vi "Object_Create.vi"(0 "reference in":refnum<class "Object.lvclass">, 1 "MapRef":refnum<class "Map.lvclass">, 5 "error in (no error)":errorcluster) -> (14 "reference out":refnum<class "Object.lvclass">, 19 "error out":errorcluster)   [LabVIEW 2020, in "Object.lvclass"]
doc: "Creates an Object, and also starts a Walkabout process for every Object"
uses:
  Object.lvclass
  Map_class/Map.lvclass
  Map_class/SurfaceType.ctl
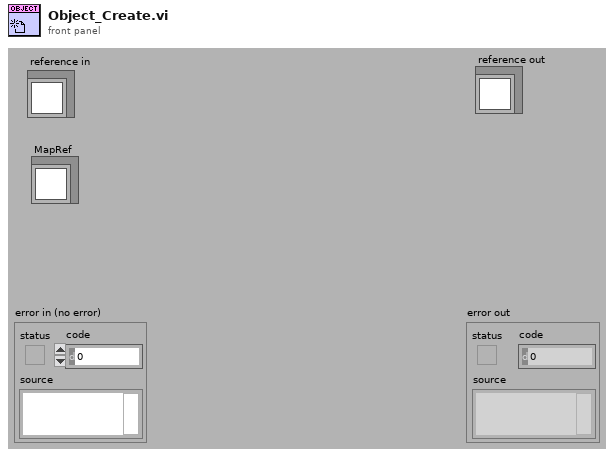
[diagram p1: front panel]
types:
  T1 = typedef "Map.lvclass/SurfaceType.ctl" = enum16{"Empty", "Wall"}
  T2 = typedef "Object.lvclass/ClassAttributes.ctl" = cluster{"Objects":i32}
  T3 = typedef "Object.lvclass/ObjectAttributes.ctl" = cluster{"X":i32, "y":i32, "Heading":enum16{"N", "E", "S", "W"}, "Map":refnum<class "Map.lvclass">, "MovementDelay":i32, "Color":u32}
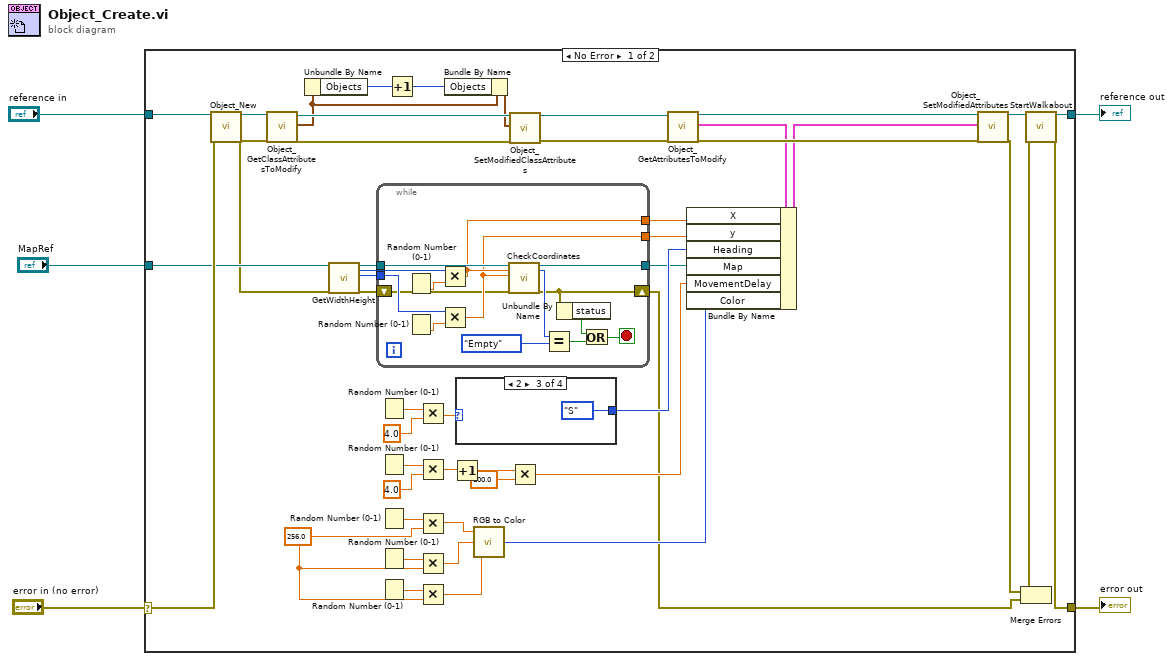
[diagram p0: block diagram]
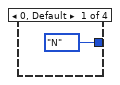
[diagram p2: hidden frame]
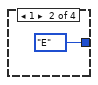
[diagram p3: hidden frame]
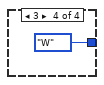
[diagram p4: hidden frame]
diagram:
  n1 = case shown="No Error" "error in (no error)" {
    selector: "error in (no error)" -> [w53 w74]
    tunnel: [w45 w74] -> w5
    tunnel: "reference in" -> [w50 w73]
    tunnel: [w47 w73] -> w3
    tunnel: "MapRef" -> [w16 _]
    frame No Error {
      w24 = 256.0 ("y")
      n2 = call "Object_New.vi"("reference in"=w50, "error in (no error)"=w53) -> ("reference out"=w15:refnum<class "Object.lvclass">, "error out"=w14:errorcluster)  [unwired: 3 in, 13 out]
      n3 = call "Object_GetClassAttributesToModify.vi"("reference in"=w15, "error in (no error)"=w14) -> ("reference out"=w13:refnum<class "Object.lvclass">, "Class attributes"=w8:T2, "error out"=w12:errorcluster)  [unwired: 1 in, 14 out]
      n4 = Unbundle By Name(w8) -> ("Objects"=w9:i32)
      n5 = call-dynamic "GetWidthHeight.vi"("reference in"=w16, "error in (no error)"=w14) -> ("reference out"=w42:refnum<class "Map.lvclass">, "Width"=w44:i32, "Height"=w43:i32, "error out"=w28:errorcluster)  [unwired: 14 out]
      n6 = while {
        tunnel: w44 -> [w72]
        tunnel: w43 -> [w69]
        tunnel: w42 -> [w68]
        tunnel: [w65] -> w41
        tunnel: [w64] -> w40
        tunnel: [w63] -> w35
        shift-right: [w61] -> w17
        shift-left: w28 -> [w62]
        stop <- w58 stop-if-true
        n7 = Random Number (0-1)() -> (number: 0 to 1=w71:dbl)
        n8 = Random Number (0-1)() -> (number: 0 to 1=w70:dbl)
        n9 = Multiply(x=w72, y=w71) -> (x*y=w65:dbl)
        n10 = Multiply(x=w69, y=w70) -> (x*y=w64:dbl)
        n11 = call-dynamic "CheckCoordinates.vi"("reference in"=w68, "X"=w65, "Y"=w64, "error in (no error)"=w62) -> ("reference out"=w63:refnum<class "Map.lvclass">, "SurfaceType"=w67:T1, "error out"=w61:errorcluster)  [unwired: 13 out]
        n12 = Equal?(x=w67, y=SurfaceType."Empty") -> (x = y?=w60:bool)
        n13 = Unbundle By Name(w61) -> ("status"=w59:bool)
        n14 = Or(x=w59, y=w60) -> (x .or. y?=w58:bool)
      }
      n15 = Random Number (0-1)() -> (number: 0 to 1=w39:dbl)
      n16 = Random Number (0-1)() -> (number: 0 to 1=w33:dbl)
      n17 = Random Number (0-1)() -> (number: 0 to 1=w27:dbl)
      n18 = Random Number (0-1)() -> (number: 0 to 1=w25:dbl)
      n19 = Random Number (0-1)() -> (number: 0 to 1=w26:dbl)
      n20 = Increment(x=w9) -> (x+1=w6:i32)
      n21 = Multiply(x=w39, y=4.0) -> (x*y=w37:dbl)
      n22 = Multiply(x=w33, y=4.0) -> (x*y=w32:dbl)
      n23 = Multiply(x=w27, y=w24) -> (x*y=w23:dbl)
      n24 = Multiply(x=w25, y=w24) -> (x*y=w22:dbl)
      n25 = Multiply(x=w26, y=w24) -> (x*y=w21:dbl)
      n26 = Bundle By Name(cluster=w8, "Objects"=w6) -> (w7:T2)
      n27 = Increment(x=w32) -> (x+1=w31:dbl)
      n28 = case shown="2" w37 {
        tunnel: [enum16{"N", "E", "S", "W"}."N" ("Heading") enum16{"N", "E", "S", "W"}."E" ("Heading") enum16{"N", "E", "S", "W"}."S" ("Heading") enum16{"N", "E", "S", "W"}."W" ("Heading")] -> w36
        frame 0, Default {
        }
        frame 1 {
        }
        frame 2 {
        }
        frame 3 {
        }
      }
      n29 = call <vilib>:"RGB to Color.vi"("B"=w21, "G"=w22, "R"=w23) -> ("Color"=w20:u32)
      n30 = call "Object_SetModifiedClassAttributes.vi"("reference in"=w13, "Class attributes"=w7, "error in (no error)"=w12) -> ("reference out"=w11:refnum<class "Object.lvclass">, "error out"=w10:errorcluster)  [unwired: 2 in, 13 out]
      n31 = Multiply(x=w31, y=100.0) -> (x*y=w29:dbl)
      n32 = call "Object_GetAttributesToModify.vi"("reference in"=w11, "error in (no error)"=w10) -> ("reference out"=w51:refnum<class "Object.lvclass">, "Attributes"=w19:T3, "error out"=w52:errorcluster)  [unwired: 1 in, 14 out]
      n33 = Bundle By Name(cluster=w19, "X"=w41, "y"=w40, "Heading"=w36, "Map"=w35, "MovementDelay"=w29, "Color"=w20) -> (w18:T3)
      n34 = call "Object_SetModifiedAttributes.vi"("reference in"=w51, "Attributes"=w18, "error in (no error)"=w52) -> ("reference out"=w48:refnum<class "Object.lvclass">, "error out"=w49:errorcluster)  [unwired: 3 in, 12 out]
      n35 = Merge Errors(w49, w17) -> (w46:errorcluster)
      n36 = call "StartWalkabout.vi"("reference in"=w48, "error in (no error)"=w46) -> ("reference out"=w47:refnum<class "Object.lvclass">, "error out"=w45:errorcluster)  [unwired: 1 in, 15 out]
    }
    frame Error {
    }
  }
  "error out" <- w5
  "reference out" <- w3
